vi "Stop.vi"(8 "error in (no error)":errorcluster, 11 "Protected Actor Handle in":refnum<class "Protected Actor Handle.lvclass">) -> (0 "error out":errorcluster)   [LabVIEW 2020, in "Actor Framework.lvlib" / "Protected Actor Handle.lvclass"]
doc: "Sends the Stop Msg to the actor with normal priority."
uses:
  Protected Actor Handle.lvclass
  Stop Msg/Stop Msg.lvclass
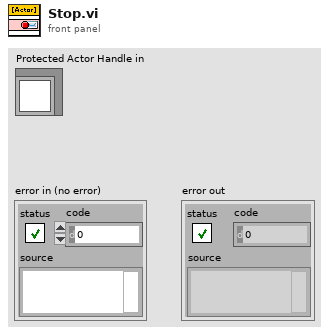
[diagram p1: front panel]
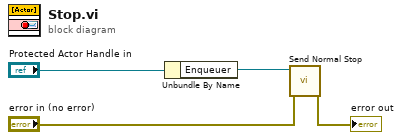
[diagram p0: block diagram]
diagram:
  n1 = Unbundle By Name("Protected Actor Handle in") -> ("Enqueuer"=w3:refnum<class "Message Enqueuer.lvclass">)
  n2 = call "Send Normal Stop.vi"("error in (no error)"="error in (no error)", "Message Enqueuer"=w3) -> ("error out"=→"error out":errorcluster)  [unwired: 9 in]
